vi "_083.vi"() -> ()   [LabVIEW 2024]
panel:
  out "appended array":i32[](array[numeric])
  out "sorted array 3":i32[](array[numeric])
  out "sorted array 2":i32[](array[numeric])
  out "first subarray":i32[](array[numeric])
  out "second subarray":i32[](array[numeric])
  out "sorted array":i32[](array[numeric])
  # "Fundamentals :"
  # "12~>After running this VI,what is the value displayed in the o/p & iteration count?"
  # "Nrml Approach :"
  # "Dfrnt Approach :"
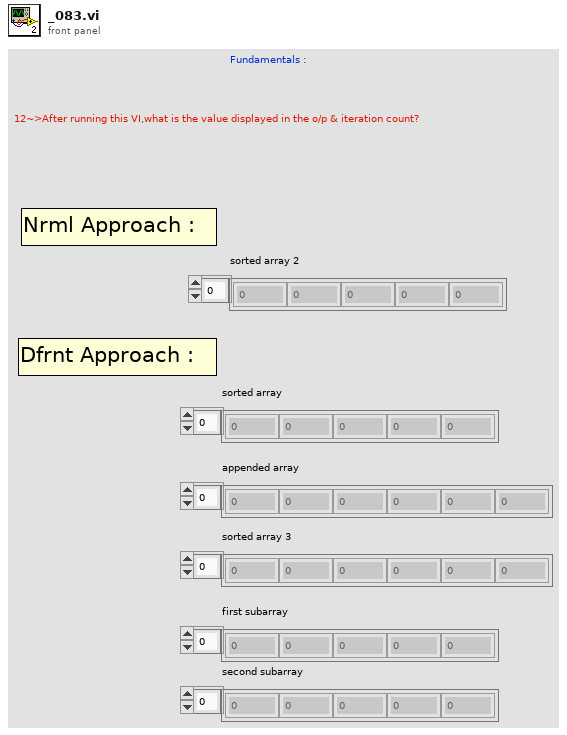
[diagram p1: front panel]
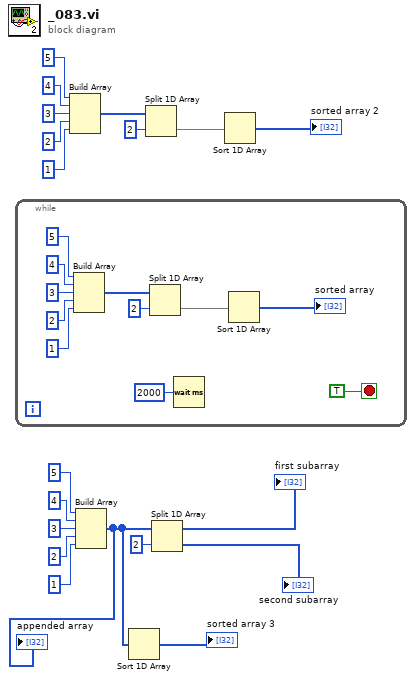
[diagram p0: block diagram]
diagram:
  n1 = while {
    stop <- TRUE stop-if-true
    n2 = Build Array "Build Array"(5, 4, 3, 2, 1) -> (w25:i32[])
    n3 = Split 1D Array(array=w25, index=2) -> (second subarray=w23:i32[])  [unwired: 1 out]
    n4 = Wait (ms)(milliseconds to wait=u32 2000) -> ()  [unwired: 1 out]
    n5 = Sort 1D Array(array=w23) -> (sorted array=→"sorted array":i32[])
  }
  n6 = Build Array "Build Array"(5, 4, 3, 2, 1) -> (w6:i32[])
  n7 = Build Array "Build Array"(5, 4, 3, 2, 1) -> (w1:i32[])
  "appended array" <- w1
  n8 = Sort 1D Array(array=w1) -> (sorted array=→"sorted array 3":i32[])
  n9 = Split 1D Array(array=w6, index=2) -> (second subarray=w4:i32[])  [unwired: 1 out]
  n10 = Split 1D Array(array=w1, index=2) -> (first subarray=→"first subarray":i32[], second subarray=→"second subarray":i32[])
  n11 = Sort 1D Array(array=w4) -> (sorted array=→"sorted array 2":i32[])
